vi "Copy_Proj_Data.vi"(8 "error in (no error)":errorcluster, 9 "IB_Destination.lvclass":refnum<class "IB_Destination.lvclass">, 10 "IB_Tree_Item_Proj in":refnum<class "IB_Tree_Item_Proj.lvclass">, 11 "IB_Source_Container in":refnum<class "IB_Source_Container.lvclass">) -> (0 "error out":errorcluster, 3 "IB_Source_Container out":refnum<class "IB_Source_Container.lvclass">)   [LabVIEW 2020, in "IB_Source_Container.lvclass"]
uses:
  <vilib>/AppBuilder/IB_Classes/Source/Container/IB_Source_Container.lvclass
  <vilib>/AppBuilder/IB_Classes/Source/Container/IB_Source_Container.lvclass/IB_Source_Container.ctl
  <vilib>/AppBuilder/IB_Classes/Tree_Item_Proj_Container/IB_Tree_Item_Proj_Container.lvclass
  <vilib>/AppBuilder/IB_Classes/Tree_Item_Proj_Contained_File/IB_Tree_Item_Proj_Contained_File.lvclass
  <vilib>/AppBuilder/IB_Classes/Source/File/CtrFile/IB_CtrFile.lvclass
  <vilib>/AppBuilder/IB_Classes/Tree_Item_Proj/IB_Tree_Item_Proj.lvclass
  <vilib>/AppBuilder/IB_Classes/Source/IB_Source.lvclass
  e:/builds/penguin/labview/branches/2020/dev/dist/vi.lib/AppBuilder/IB_Classes/Tree_Item_Proj/IB_Tree_Item_Proj.lvclass
  e:/builds/penguin/labview/branches/2020/dev/dist/vi.lib/AppBuilder/IB_Classes/Tree_Item/IB_Tree_Item.lvclass
  e:/builds/penguin/labview/branches/2020/dev/dist/vi.lib/AppBuilder/IB_Classes/Tree_Item_Proj_Container/IB_Tree_Item_Proj_Container.lvclass
  <vilib>/AppBuilder/IB_Classes/Destination/IB_Destination.lvclass
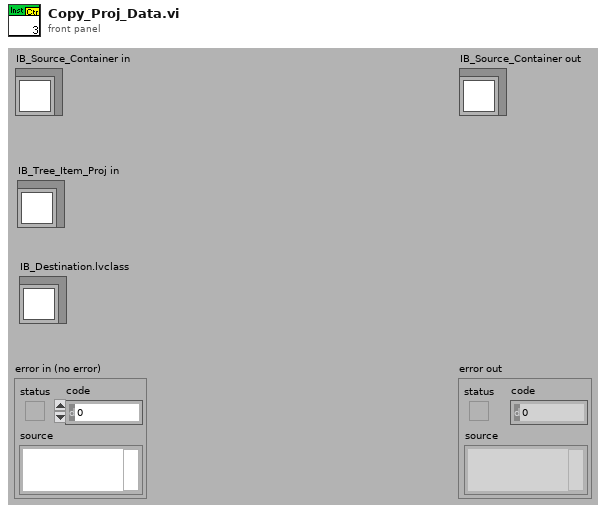
[diagram p1: front panel]
types:
  T1 = typedef "IB_Tree_Item_Proj.ctl" = cluster{"itemID":string, "path":path}
  T2 = typedef "IB_Tree_Item_Proj_Container.ctl" = cluster{"ctr files":refnum<class "IB_Tree_Item_Proj_Contained_File.lvclass">[], "previewed?":bool, "expanded?":bool, "preview error?":bool}
  T3 = typedef "IB_CtrFile.ctl" = cluster{"parentTag":string, "force save?":bool}
  T4 = typedef "IB_Source_Container.ctl" = cluster{"files":refnum<class "IB_CtrFile.lvclass">[], "previewed?":bool, "preview error?":bool}
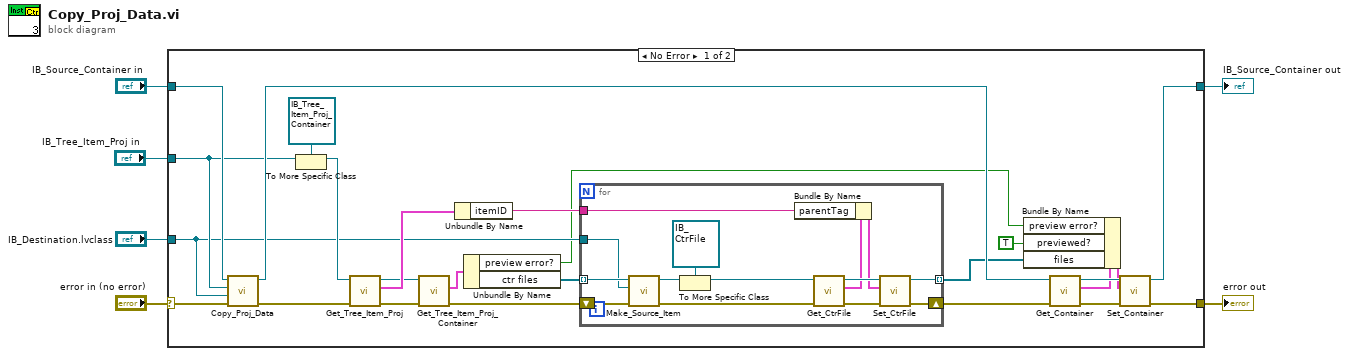
[diagram p0: block diagram]
diagram:
  n1 = case shown="No Error" "error in (no error)" {
    selector: "error in (no error)" -> [w30 w46]
    tunnel: [w27 w46] -> w6
    tunnel: [w24 w47] -> w5
    tunnel: "IB_Tree_Item_Proj in" -> [w19 _]
    tunnel: "IB_Source_Container in" -> [w31 w47]
    tunnel: "IB_Destination.lvclass" -> [w10 _]
    frame No Error {
      n2 = call-parent "Copy_Proj_Data.vi"("error in (no error)"=w30, "IB_Destination.lvclass"=w10, "IB_Tree_Item_Proj in"=w19, "IB_Source in"=w31) -> ("error out"=w12:errorcluster, "IB_Source out"=w25:refnum<class "IB_Source_Container.lvclass">)  [unwired: 6 out]
      n3 = To More Specific Class(target class=refnum<class "IB_Tree_Item_Proj_Container.lvclass"> refnum ("IB_Tree_Item_Proj_Container.lvclass"), reference=w19) -> (specific class reference=w14:refnum<class "IB_Tree_Item_Proj_Container.lvclass">)  [unwired: 1 in, 1 out]
      n4 = call <vilib>:"Get_Tree_Item_Proj.vi"("error in (no error)"=w12, "IB_TreeProjectItem in"=w14) -> ("error out"=w11:errorcluster, "data"=w16:T1, "IB_TreeProjectItem out"=w13:refnum<class "IB_Tree_Item_Proj_Container.lvclass">)  [unwired: 7 out]
      n5 = call <vilib>:"Get_Tree_Item_Proj_Container.vi"("error in (no error)"=w11, "IB_Tree_Item_Proj_Container in"=w13) -> ("error out"=w9:errorcluster, "data"=w29:T2)  [unwired: 8 out]
      n6 = Unbundle By Name(w16) -> ("itemID"=w15:string)
      n7 = Unbundle By Name(w29) -> ("preview error?"=w7:bool, "ctr files"=w20:refnum<class "IB_Tree_Item_Proj_Contained_File.lvclass">[])
      n8 = for {
        tunnel: w20 -> [w45] mode=indexing
        tunnel: [w42] -> w17 mode=indexing
        tunnel: w15 -> [w32]
        tunnel: w10 -> [w41]
        shift-right: [w39] -> w8
        shift-left: w9 -> [w40]
        n9 = call-dynamic "Make_Source_Item.vi"("error in (no error)"=w40, "IB_Destination.lvclass"=w41, "IB_Tree_Item_Proj_Contained_File in"=w45) -> ("error out"=w36:errorcluster, "IB_Source.lvclass"=w43:refnum<class "IB_Source.lvclass">)  [unwired: 7 out]
        n10 = To More Specific Class(target class=refnum<class "IB_CtrFile.lvclass"> refnum ("IB_CtrFile.lvclass"), reference=w43) -> (specific class reference=w38:refnum<class "IB_CtrFile.lvclass">)  [unwired: 1 in, 1 out]
        n11 = call <vilib>:"Get_CtrFile.vi"("error in (no error)"=w36, "IB_CtrFile in"=w38) -> ("error out"=w35:errorcluster, "parentTag"=w34:T3, "IB_CtrFile out"=w37:refnum<class "IB_CtrFile.lvclass">)  [unwired: 7 out]
        n12 = Bundle By Name(cluster=w34, "parentTag"=w32) -> (w33:T3)
        n13 = call <vilib>:"Set_CtrFile.vi"("error in (no error)"=w35, "parentTag"=w33, "IB_CtrFile in"=w37) -> ("error out"=w39:errorcluster, "IB_CtrFile out"=w42:refnum<class "IB_CtrFile.lvclass">)  [unwired: 7 out]
      }
      n14 = call <vilib>:"Get_Container.vi"("error in (no error)"=w8, "IB_Source_Container in"=w25) -> ("error out"=w28:errorcluster, "data"=w23:T4, "IB_Source_Container out"=w26:refnum<class "IB_Source_Container.lvclass">)  [unwired: 7 out]
      n15 = Bundle By Name(cluster=w23, "preview error?"=w7, "previewed?"=TRUE, "files"=w17) -> (w22:T4)
      n16 = call <vilib>:"Set_Container.vi"("error in (no error)"=w28, "data"=w22, "IB_Source_Container in"=w26) -> ("error out"=w27:errorcluster, "IB_Source_Container out"=w24:refnum<class "IB_Source_Container.lvclass">)  [unwired: 7 out]
    }
    frame Error {
    }
  }
  "error out" <- w6
  "IB_Source_Container out" <- w5
